vi "SS2 Live_Gate Data Q.vi"(5 "error in (no error)":errorcluster, 6 "SS2 Live Gate Data Q Name":string="SS2 Live Gate Data Q") -> (1 "error out":errorcluster, 2 "SS2 Live Gate Data Q":refnum<queue>)   [LabVIEW 2019]
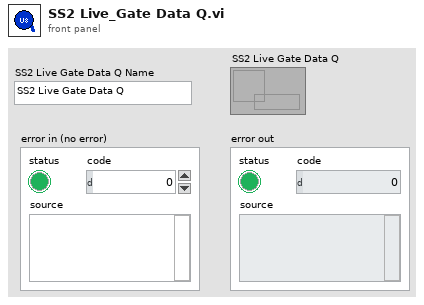
[diagram p1: front panel]
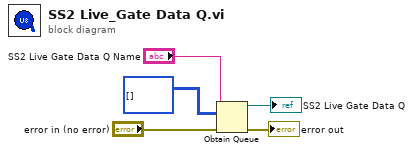
[diagram p0: block diagram]
diagram:
  n1 = Obtain Queue(name (unnamed)="SS2 Live Gate Data Q Name", element data type=u8[][] [] ("second subarray"), error in (no error)="error in (no error)") -> (queue out=→"SS2 Live Gate Data Q":refnum<queue>, error out=→"error out":errorcluster)  [unwired: 2 in, 1 out]
